vi "SV TDMS Read Order Level Components (1xM).vi"(0 "tdms file":refnum<k34>, 5 "group name in":string, 7 "channel names in":string[](array[string]), 11 "error in":errorcluster) -> (3 "scale labels":T1, 4 "tdms file out":refnum<k34>, 6 "group name out":string, 8 "channel names out":string[](array[string]), 10 "order components":cluster{"X":dbl[], "Y":dbl[]}[](array[cluster]), 13 "spectrum info":T2 {"x-axis units" items=["Time (s)"=0, "Frequency-CB (Hz)"=1, "Frequency-CPB (Hz)"=1248, "Frequency-Arbitrary (Hz)"=2357, "Quefrency (s)"=2, "Revolutions (rev)"=3, "Order"=4, "Speed (RPM)"=11, "Speed (rad/s)"=21, "Index"=65535]; "weighting filter" items=["Linear", "A-weighting", "B-weighting", "C-weighting", "ITU-R 468-4", "Dolby", "CCITT", "C-message", "Wb", "Wc", "Wd", "We", "Wf", "Wh", "Wj", "Wk", "Wm", "AES17 20 kHz lowpass", "AES17 40 kHz lowpass", "AES17 20 kHz highpass", "AES17 40 kHz highpass"]; "dB reference [EU]" format="%.2f"; "engineering units" items=["custom..."=0, "V"=1, "A"=21, "C"=30, "pC"=31, "s"=32, "-"=29, "Pa"=2, "N"=20, "g"=3, "m/s^2"=4, "m/s"=5, "m"=6, "mm/s"=12, "mm"=13, "micron/s"=14, "micron"=15, "in/s^2"=7, "in/s"=8, "in"=9, "mil/s"=10, "mil"=11, "rad/s^2"=16, "rad/s"=17, "rad"=18, "deg/s^2"=26, "deg/s"=27, "deg"=28, "RPM"=22, "cycle/s^2"=23, "Hz"=24, "cycle"=25, "strain"=19]; "spectral info"."window" items=["None "=0, "Hanning"=1, "Hamming"=2, "Blackman-Harris"=3, "Exact Blackman"=4, "Blackman"=5, "Flat Top"=6, "4 Term B-Harris "=7, "7 Term B-Harris"=8, "Low Sidelobe"=9, "Force - Exponential"=10, "Gaussian"=62]}, 15 "error out":errorcluster)   [LabVIEW 2017]
doc: "Reads the specified .tdms file and returns data in a format specific to the polymorphic instance selected."
uses:
  <vilib>/addons/_NISVFA/_Shared subVIs/Controls/svc_Spectrum Info.ctl
  <vilib>/addons/_NISVFA/_Shared subVIs/Controls/svc_X-Axis Units.ctl
  <vilib>/addons/_NISVFA/_Shared subVIs/Controls/svc_Spectrum Type.ctl
  <vilib>/addons/_NISVFA/_Shared subVIs/Controls/svc_Engineering Units Text Ring.ctl
  <vilib>/addons/_NISVFA/_Shared subVIs/Controls/svc_Weighting Filter Text Ring.ctl
  <vilib>/addons/_NISVFA/_Shared subVIs/Controls/svc_Complimentary Spectrum Units.ctl
  <vilib>/addons/_NISVFA/_Shared subVIs/Controls/NI Channel Properties.ctl
  <vilib>/addons/_NISVFA/_Shared subVIs/Controls/SV Channel Properties.ctl
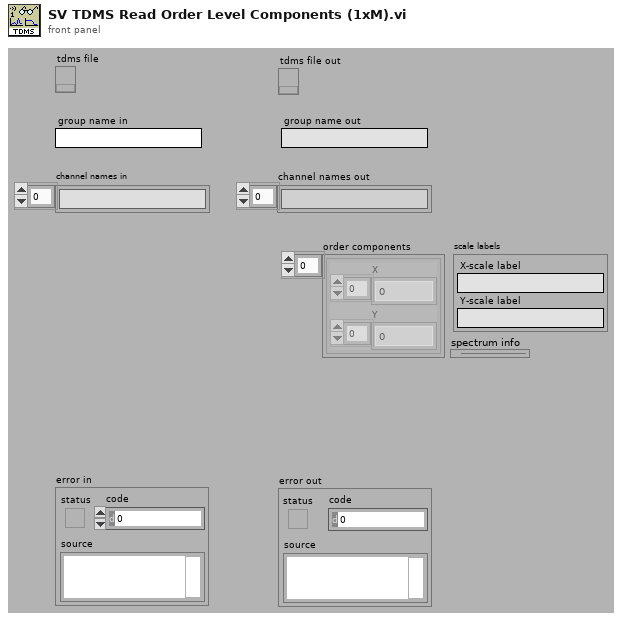
[diagram p1: front panel]
types:
  T1 = cluster{"X-scale label":string, "Y-scale label":string}
  T2 = typedef "svc_Spectrum Info.ctl" = cluster{"channel name":string, "description":string, "x-axis units":T3, "spectral info":cluster{"spectrum type":T4, "linear/dB":enum16{"linear", "dB"}, "window":u16, "window size":i32, "FFT size":i32}, "engineering units":T5, "custom label":string, "dB reference [EU]":dbl, "peak units":enum16{"rms", "peak", "peak-peak"}, "weighting filter":T6, "spectral density?":bool, "unit label":string, "spectrum skewed?":bool, "complimentary spectrum units":T7}
  T3 = typedef "svc_X-Axis Units.ctl" = u16
  T4 = typedef "svc_Spectrum Type.ctl" = enum16{"FFT Spectrum [complex]", "Amplitude [Magnitude]", "Power [Magnitude^2]", "Cross Spectrum [complex]", "Frequency Response [Complex]"}
  T5 = typedef "svc_Engineering Units Text Ring.ctl" = u16
  T6 = typedef "svc_Weighting Filter Text Ring.ctl" = u16
  T7 = typedef "svc_Complimentary Spectrum Units.ctl" = enum16{"none", "radians", "degrees", "cycles", "imaginary"}
  T8 = typedef "SV Channel Properties.ctl" = u16
  T9 = typedef "NI Channel Properties.ctl" = u16
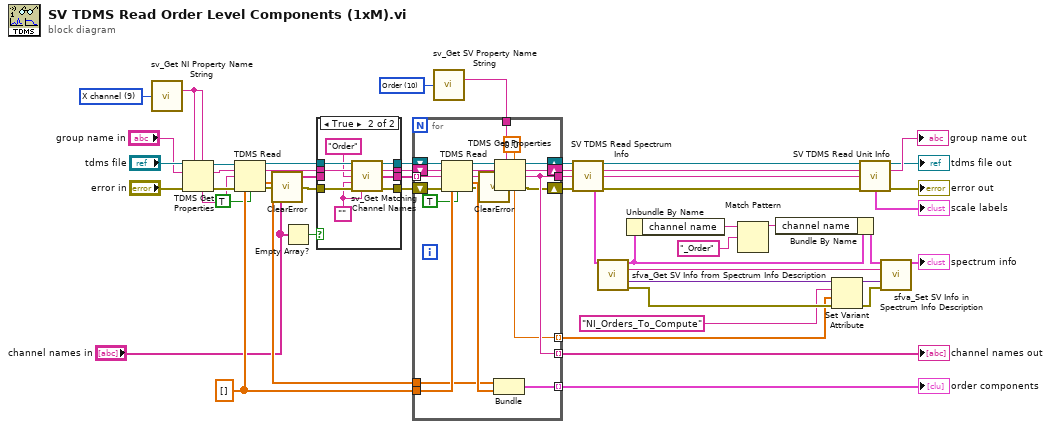
[diagram p0: block diagram]
diagram:
  w18 = T8 10 items=["Engineering units", "Custom unit label", "Weighting filter", "Pregain", "Octave standard", "Octave bandwidth", "Octave low band", "Octave high band", "Spectrum skewed", "Samples / revolution", "Order"] ("property")
  w52 = T9 9 items=["Channel name", "Channel description", "Y-axis label", "Y-axis unit string", "X-axis label", "X-axis unit string", "x0", "dx", "Number of samples", "X channel", "Filter settled", "dB reference", "Window", "Window parameter", "Window size", "FFT size", "Peak units", "Spectrum type", "Magnitude scale", "Spectral density", "Sensor sensitivity (mV/EU)", "X-axis domain", "LabVIEW datatype"] ("property")
  w48 = dbl[] [] ("X")
  n1 = call <vilib>:"sv_Get NI Property Name String.vi"("property"=w52) -> ("TDMS property name"=w43:string)  [unwired: 13 in, 1 out]
  n2 = TDMS Get Properties(5:w43, 7:w43, 8:"error in", 10:"group name in", 11:"tdms file") -> (0:w50:errorcluster, 2:w49:string, 3:w45:refnum<k34>, 4:w41:string)  [unwired: 1 in, 2 out]
  n3 = TDMS Read(0:w45, 5:w49, 7:w41, 11:w50, 12:w48, 13:TRUE ("return channels in file order? (F)")) -> (4:w40:refnum<k34>, 6:w39:string, 10:w47:dbl[], 15:w2:errorcluster)  [unwired: 2 in, 2 out]
  n4 = call <vilib>:"ClearError.vi"("error in (no error)"=w2) -> ("error out"=w38:errorcluster)
  n5 = Empty Array?(array="channel names in") -> (empty?=w33:bool)
  n6 = case shown="True" w33 {
    tunnel: w40 -> [w56 w65]
    tunnel: w39 -> [w55 w64]
    tunnel: w38 -> [w53 w63]
    tunnel: [w53 w62] -> w37
    tunnel: [w55 w61] -> w36
    tunnel: [w56 w60] -> w35
    tunnel: [w54 w59] -> w34
    tunnel: "channel names in" -> [w54 _]
    frame False {
    }
    frame True {
      w57 = ""
      n7 = call <vilib>:"sv_Get Matching Channel Names.vi"("tdms file"=w65, "group name"=w64, "channel name substring"="Order" ("channel name"), "channel name substring2"=w57, "error in (no error)"=w63, "separator"=w57) -> ("tdms file out"=w60:refnum<k34>, "group name out"=w61:string, "channel names"=w59:string[], "error out"=w62:errorcluster)  [unwired: 6 in]
    }
  }
  n8 = call <vilib>:"sv_Get SV Property Name String.vi"("property"=w18) -> ("TDMS property name"=w17:string)  [unwired: 13 in, 1 out]
  n9 = for {
    shift-right: [w75] -> w25
    shift-left: w35 -> [w86]
    shift-right: [w72] -> w23
    shift-left: w37 -> [w84]
    tunnel: w48 -> [w83]
    tunnel: [w81] -> w51 mode=indexing
    shift-right: [w74] -> w24
    shift-left: w36 -> [w85]
    tunnel: w47 -> [w80]
    tunnel: w34 -> [w79] mode=indexing
    tunnel: [w73] -> w27 mode=indexing
    tunnel: [w73] -> w26
    tunnel: w17 -> [w70]
    tunnel: [w68] -> w13 mode=indexing
    n10 = TDMS Read(0:w86, 5:w85, 7:w79, 11:w84, 12:w83, 13:TRUE ("return channels in file order? (F)")) -> (4:w76:refnum<k34>, 6:w77:string, 8:w78:string, 10:w82:dbl[], 15:w67:errorcluster)  [unwired: 2 in, 1 out]
    n11 = call <vilib>:"ClearError.vi"("error in (no error)"=w67) -> ("error out"=w71:errorcluster)
    n12 = Bundle("X"=w80, "X"=w82) -> (w81:cluster{"X":dbl[], "X":dbl[]})  [unwired: 1 in]
    n13 = TDMS Get Properties(5:0.0 ("x"), 7:w70, 8:w71, 9:w78, 10:w77, 11:w76) -> (0:w72:errorcluster, 1:w73:string, 2:w74:string, 3:w75:refnum<k34>, 4:w68:dbl)  [unwired: 1 out]
  }
  "order components" <- w51
  "channel names out" <- w27
  n14 = call <vilib>:"SV TDMS Read Spectrum Info.vi"("tdms file"=w25, "group name in"=w24, "channel name in"=w26, "error in"=w23) -> ("tdms file out"=w28:refnum<k34>, "group name out"=w29:string, "channel name out"=w30:string, "spectrum info"=w12:T2, "error out"=w31:errorcluster)  [unwired: 7 in]
  n15 = call <vilib>:"sfva_Get SV Info from Spectrum Info Description.vi"("spectrum info"=w12) -> ("spectrum info"=w7:T2, "description"=w11:string, "SV Info"=w15:variant, "error out"=w16:errorcluster)  [unwired: 10 in, 1 out]
  n16 = Unbundle By Name(w7) -> ("channel name"=w5:string)
  n17 = Match Pattern(string=w5, regular expression="_Order") -> (before substring=w4:string)  [unwired: 1 in, 3 out]
  n18 = Bundle By Name(cluster=w7, "channel name"=w4) -> (w6:T2)
  n19 = Set Variant Attribute(Variant=w15, name="NI_Orders_To_Compute", value=w13, error in=w16) -> (Variant out=w10:variant, error out=w9:errorcluster)  [unwired: 1 out]
  n20 = call <vilib>:"SV TDMS Read Unit Info.vi"("tdms file"=w28, "group name"=w29, "channel name"=w30, "error in (no error)"=w31) -> ("tdms file out"=→"tdms file out":refnum<k34>, "group name out"=→"group name out":string, "scale labels"=→"scale labels":T1, "error out"=→"error out":errorcluster)  [unwired: 6 in, 2 out]
  n21 = call <vilib>:"sfva_Set SV Info in Spectrum Info Description.vi"("spectrum info"=w6, "description"=w11, "SV Info"=w10, "error in (no error)"=w9) -> ("spectrum info"=→"spectrum info":T2)  [unwired: 10 in, 1 out]
